vi "Write Digital Port.vi"(8 "error in (no error)":errorcluster, 10 "Boolean":bool, 11 "Digital Output in":refnum<class "Digital Output.lvclass">) -> (0 "error out":errorcluster, 3 "Digital Output out":refnum<class "Digital Output.lvclass">)   [LabVIEW 2021, in "Interface.lvlib" / "Digital Output.lvclass"]
uses:
  Digital Output.lvclass
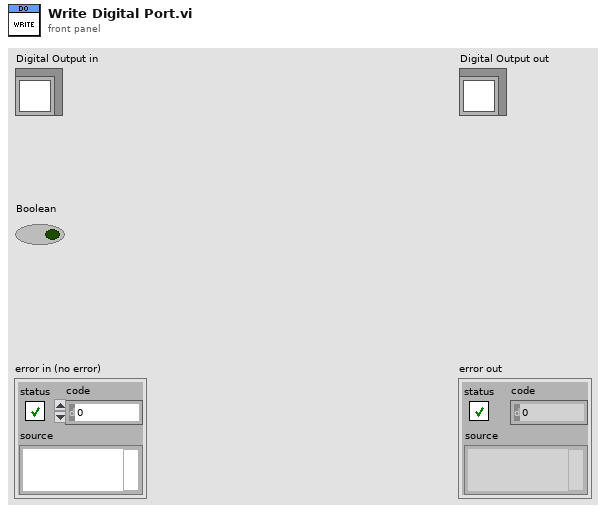
[diagram p1: front panel]
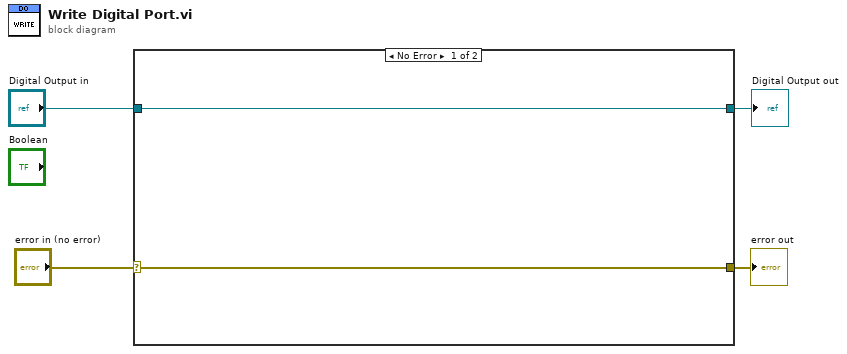
[diagram p0: block diagram]
diagram:
  n1 = case shown="No Error" "error in (no error)" {
    selector: "error in (no error)" -> [w5 w8]
    tunnel: [w5 w8] -> w3
    tunnel: [w6 w7] -> w1
    tunnel: "Digital Output in" -> [w6 w7]
    frame No Error {
    }
    frame Error {
    }
  }
  "error out" <- w3
  "Digital Output out" <- w1
